vi "EAGLE Setup Screen V1.vi"() -> ()   [LabVIEW 2015]
panel:
  in  "AvgPulse":dbl(slide)=1.0 caption="Average Pulse\nEnergy [mJ]" min=0.0 max=1.0 step=0.1 scale=0.0..1.0
  out "Table Control":string[][](table)
  in  "EyeColor":enum32{"Dark", "Blue/Green"}(radio) caption="Eye Color"
  in  "EyeSelect":enum32{"Right Eye", "Left Eye"}(radio) caption="Treated Eye"
  in  "DisFromLimbus":dbl(slide)=1.0 caption="Distance From \nLimbus [um]" min=0.0 max=1.0 step=0.1 scale=0.0..1.0
  in  "TBetweenPulses":u8(slide)=4 caption="Time Between \nPulses [mSec]" min=4 max=10 step=1 scale=4.0..10.0
  in  "LaserShots":u8(slide)=1 caption="Number of \nLaser Shots" min=1 max=100 step=1 scale=1.0..100.0
  in  "ID":string caption="Patient ID"
  in  "TreatArea":enum32{"Upper 180", "Lower 180", "Full 360"}(radio) caption="Treatment Area"
  in  "SaveAs":bool
  in  "Save":bool
  in  "FillSetupList":bool
  in  "Treatment Setup":string(combo)
  in  "Done":bool
  # "Treatment Info"
  # "Patient Info"
  # "Treatment Summery"
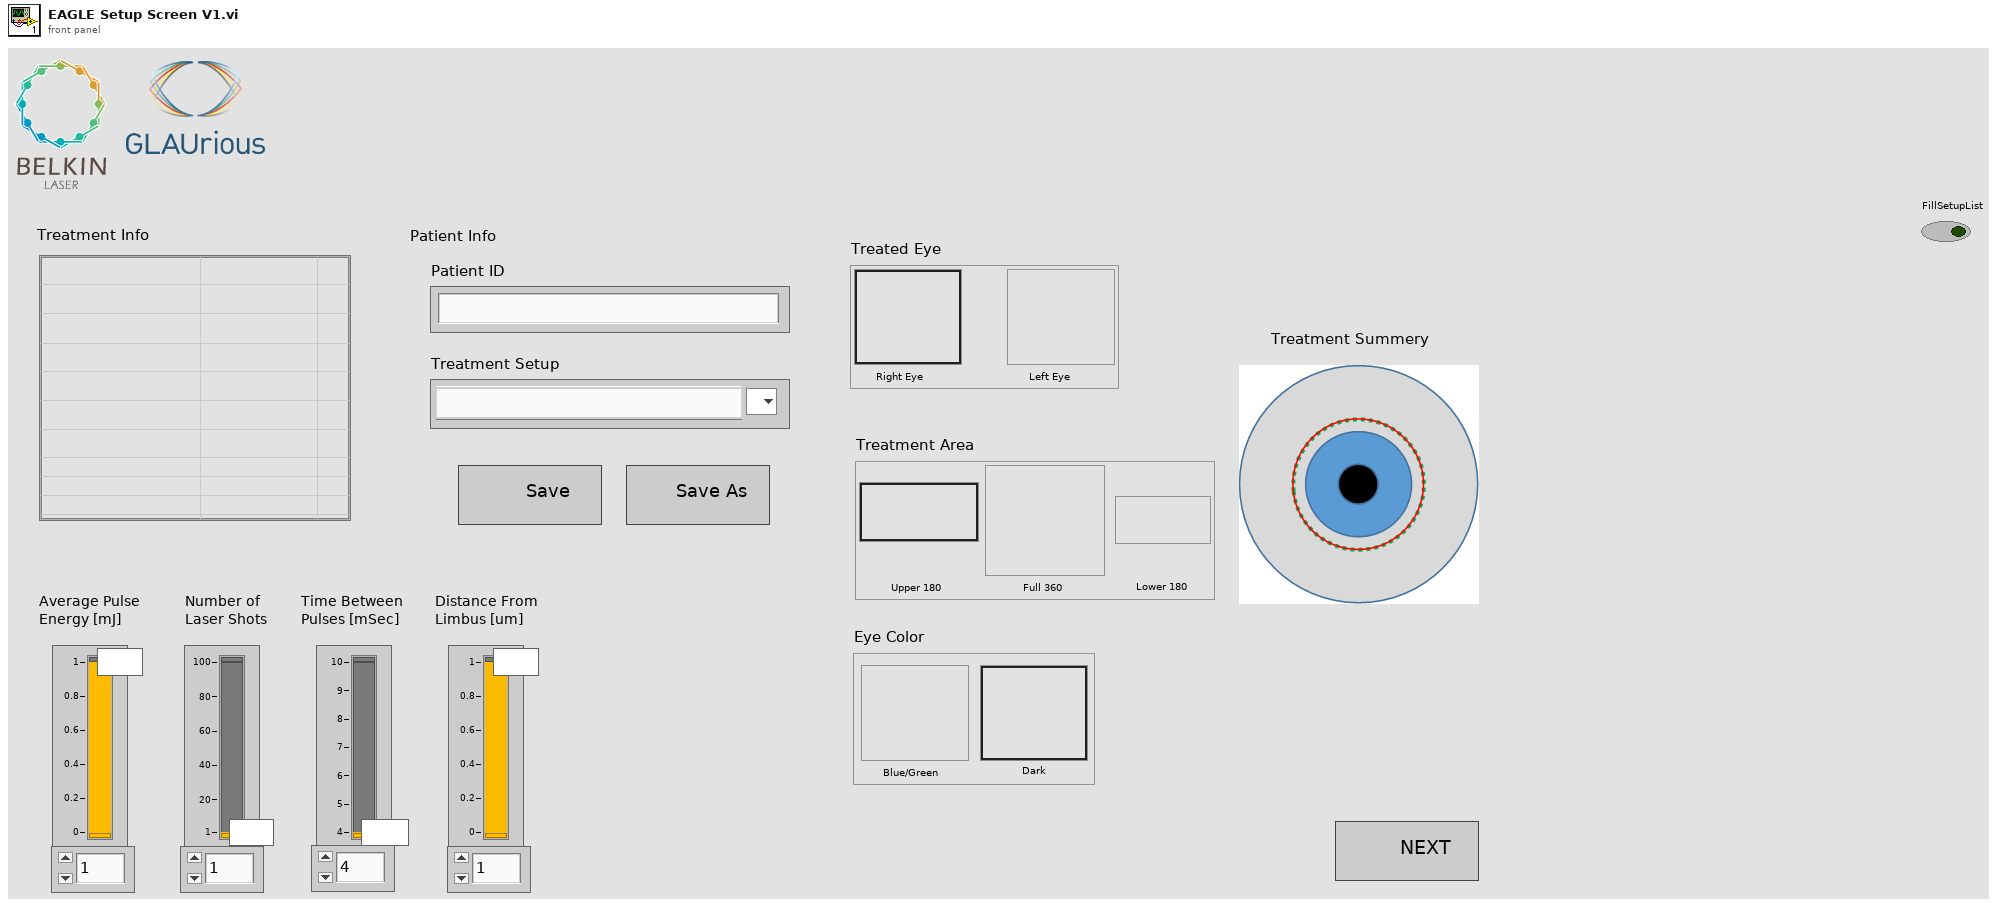
[diagram p1: front panel]
types:
  T1 = cluster{"EyeSelect":enum32{"Right Eye", "Left Eye"}, "TBetweenPulses":u8, "LaserShots":u8, "TreatArea":enum32{"Upper 180", "Lower 180", "Full 360"}, "DisFromLimbus":dbl, "ID":string, "EyeColor":enum32{"Dark", "Blue/Green"}, "AvgPulse":dbl}
  T2 = typedef "LVComboBoxStrsAndValuesArrayTypeDef.ctl" = cluster{"String":string, "Value":string}[]
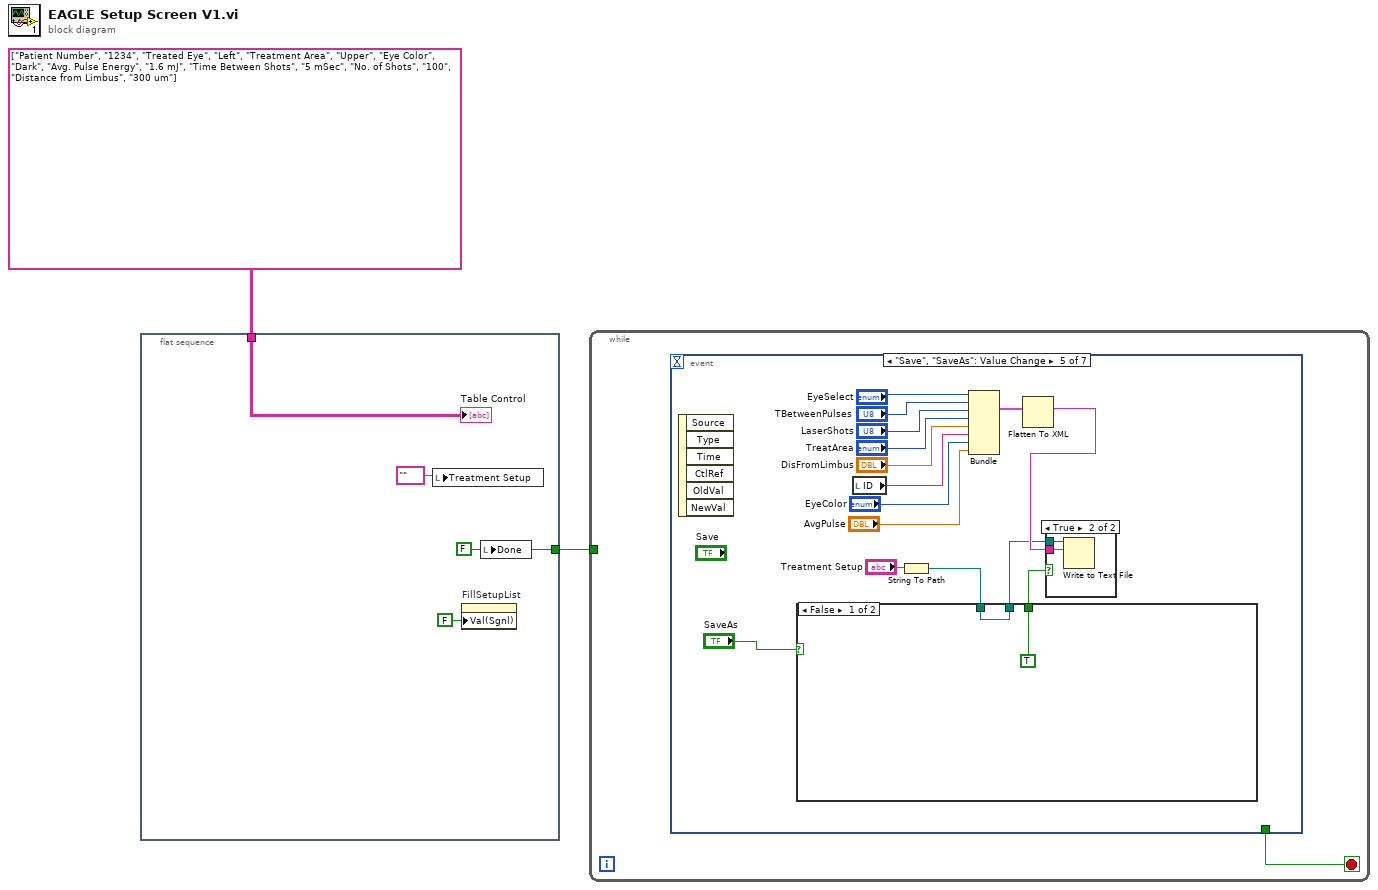
[diagram p0: block diagram]
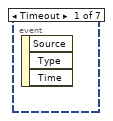
[diagram p2: hidden frame]
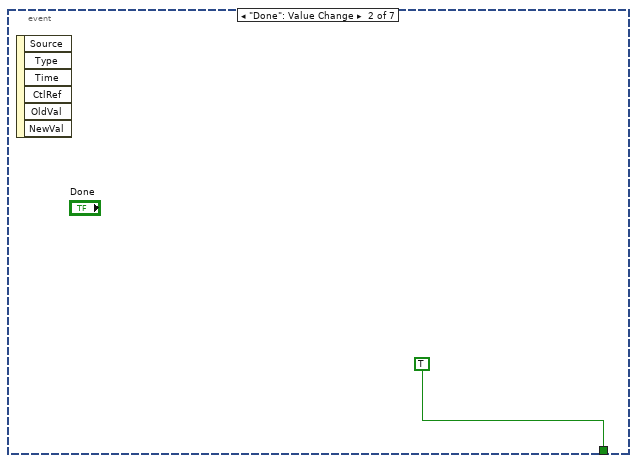
[diagram p3: hidden frame]
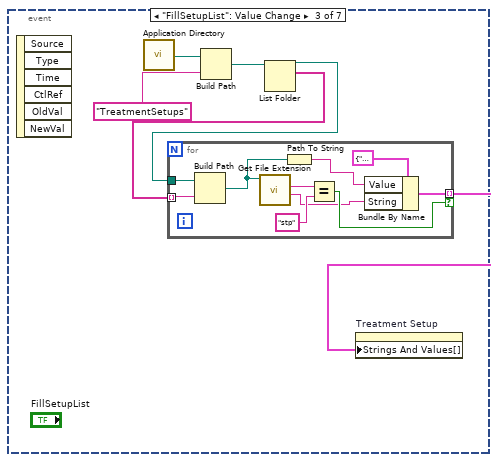
[diagram p4: hidden frame]
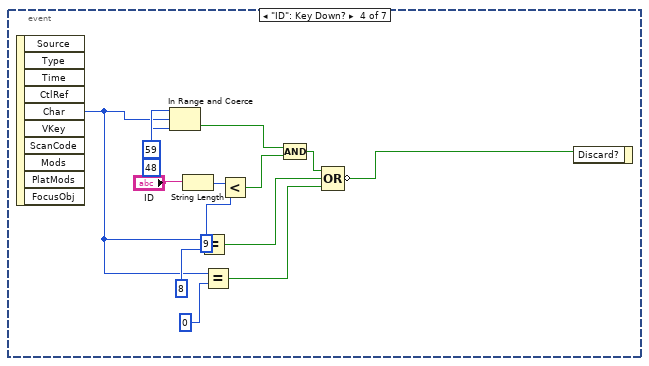
[diagram p5: hidden frame]
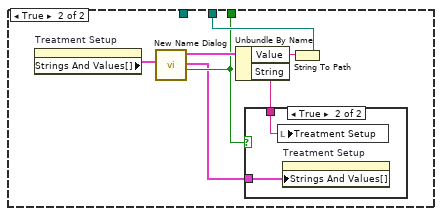
[diagram p7: hidden frame]
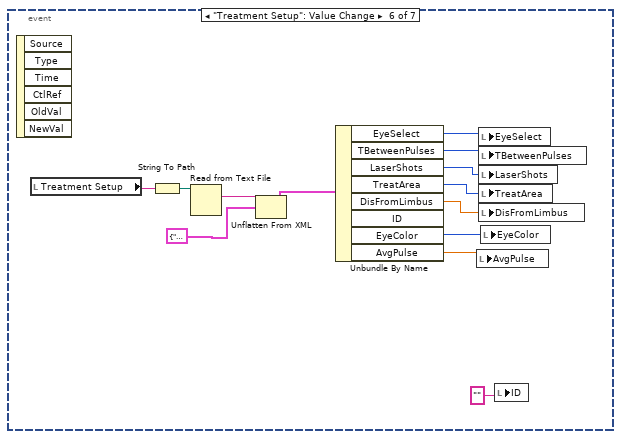
[diagram p9: hidden frame]
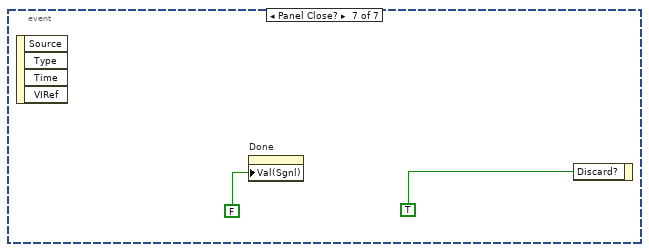
[diagram p10: hidden frame]
diagram:
  n1 = flat-sequence {
    tunnel: [w6] -> w2
    tunnel: string[][] [["Patient Number", "1234"], ["Treated Eye", "Left"], ["Treatment Area", "Upper"], ["Eye Color", "Dark"], ["Avg. Pulse Energy", "1.6 mJ"], ["Time Between Shots", "5 mSec"], ["No. of Shots", "100"], ["Distance from Limbus", "300 um"]] ("Table Control") -> [w3]
    frame #0 {
      w6 = FALSE ("Done")
      n2 = local write "Treatment Setup"("" ("Treatment Setup")) -> ()
      n3 = property on="FillSetupList" class="Bool (strict)"("Val(Sgnl)"=FALSE ("Value (Signaling)")) -> ()  [unwired: 2 in, 2 out]
      n4 = local write "Done"(w6) -> ()
      "Table Control" <- w3
    }
  }
  n5 = while {
    tunnel: w2 -> [_]
    stop <- w7 stop-if-true
    n6 = event shown="[4] \"Save\", \"SaveAs\": Value Change" {
      selector: _ -> [_ _ _ _ _ _ _]
      dyn-events: _ -> [_ _ _ _ _ _ _]
      timeout: _ -> [_ _ _ _ _ _ _]
      tunnel: [_ TRUE _ _ _ _ _] -> w7
      event Timeout {
        n7 = event-data() -> ()  [unwired: 1 in, 3 out]
      }
      event "Done": Value Change {
        n8 = event-data() -> ()  [unwired: 1 in, 6 out]
      }
      event "FillSetupList": Value Change {
        n9 = event-data() -> ()  [unwired: 1 in, 6 out]
        n10 = call <vilib>:"Application Directory.vi"() -> ("Application Directory"=w14:path)
        n11 = Build Path(base path=w14, name or relative path="TreatmentSetups") -> (appended path=w12:path)
        n12 = List Folder(path=w12) -> (path out=w10:path, filenames=w11:string[])  [unwired: 3 in, 2 out]
        n13 = for {
          tunnel: w11 -> [w19] mode=indexing
          tunnel: w10 -> [w24]
          tunnel: [w18] -> w9 mode=indexing if=w17
          n14 = Build Path(base path=w24, name or relative path=w19) -> (appended path=w22:path)
          n15 = call <vilib>:"Get File Extension.vi"("file"=w22) -> ("filename without extension"=w15:string, "lowercase file extension"=w16:string)  [unwired: 6 in, 3 out]
          n16 = Path To String(path=w22) -> (string=w20:string)
          n17 = Equal?(x=w16, y="stp") -> (x = y?=w17:bool)
          n18 = Bundle By Name(cluster=cluster{"String":string, "Value":string} {"String"="", "Value"=""}, "Value"=w20, "String"=w15) -> (w18:cluster{"String":string, "Value":string})
        }
        n19 = property on="Treatment Setup" class="CmbBox"("Strings And Values[]"=w9) -> ()  [unwired: 2 in, 2 out]
      }
      event "ID": Key Down? {
        n20 = event-data() -> ("Char"=w30:i16)  [unwired: 1 in, 9 out]
        n21 = In Range and Coerce(upper limit=i16 59, x=w30, lower limit=i16 48) -> (In Range?=w33:bool)  [unwired: 1 out]
        n22 = String Length(string="ID") -> (length=w35:i32)
        n23 = Equal?(x=w30, y=i16 8) -> (x = y?=w27:bool)
        n24 = Equal?(x=w30, y=i16 0) -> (x = y?=w26:bool)
        n25 = Less?(x=w35, y=9) -> (x < y?=w32:bool)
        n26 = Compound Arithmetic op=AND(w33, w32) -> (w28:bool)
        n27 = Compound Arithmetic op=OR(w28, w27, w26) -> (invert w25:bool)
        n28 = event-data("Discard?"=w25) -> ()  [unwired: 1 in, 1 out]
      }
      event "Save", "SaveAs": Value Change {
        n29 = event-data() -> ()  [unwired: 1 in, 6 out]
        n30 = local read "ID"() -> (w41:string)
        n31 = String To Path(string="Treatment Setup") -> (path=w44:path)
        n32 = case shown="False" "SaveAs" {
          tunnel: w44 -> [w57 _]
          tunnel: [w57 w61] -> w43
          tunnel: [TRUE w60] -> w42
          frame False {
          }
          frame True {
            n33 = property on="Treatment Setup" class="CmbBox"() -> ("Strings And Values[]"=w64:T2)  [unwired: 2 in, 2 out]
            n34 = call "New Name Dialog.vi"("Names"=w64) -> ("OK"=w60:bool, "NamesOut"=w59:cluster{"String":string, "Value":string}[], "NewName"=w63:cluster{"String":string, "Value":string})  [unwired: 8 in]
            n35 = Unbundle By Name(w63) -> ("Value"=w62:string, "String"=w58:string)
            n36 = case shown="True" w60 {
              tunnel: w59 -> [_ w66]
              tunnel: w58 -> [_ w65]
              frame False {
              }
              frame True {
                n37 = local write "Treatment Setup"(w65) -> ()
                n38 = property on="Treatment Setup" class="CmbBox"("Strings And Values[]"=w66) -> ()  [unwired: 2 in, 2 out]
              }
            }
            n39 = String To Path(string=w62) -> (path=w61:path)
          }
        }
        n40 = Bundle("EyeSelect"="EyeSelect", "TBetweenPulses"="TBetweenPulses", "LaserShots"="LaserShots", "TreatArea"="TreatArea", "DisFromLimbus"="DisFromLimbus", "ID"=w41, "EyeColor"="EyeColor", "AvgPulse"="AvgPulse") -> (w53:T1)  [unwired: 1 in]
        n41 = Flatten To XML(anything=w53) -> (xml string=w47:string)
        n42 = case shown="True" w42 {
          tunnel: w47 -> [_ w55]
          tunnel: w43 -> [_ w54]
          frame False {
          }
          frame True {
            n43 = Write to Text File(file (use dialog)=w54, text=w55) -> ()  [unwired: 2 in, 3 out]
          }
        }
      }
      event "Treatment Setup": Value Change {
        n44 = event-data() -> ()  [unwired: 1 in, 6 out]
        n45 = local read "Treatment Setup"() -> (w79:string)
        n46 = String To Path(string=w79) -> (path=w78:path)
        n47 = Read from Text File(file (use dialog)=w78) -> (text=w77:string)  [unwired: 3 in, 3 out]
        n48 = Unflatten From XML(xml string=w77, type=T1 {"EyeSelect"=enum."Right Eye", "TBetweenPulses"=0, "LaserShots"=0, "TreatArea"=enum."Upper 180", "DisFromLimbus"=0.0, "ID"="", "EyeColor"=enum."Dark", "AvgPulse"=0.0} ("output cluster")) -> (value=w76:T1)  [unwired: 1 in, 1 out]
        n49 = Unbundle By Name(w76) -> ("EyeSelect"=w75:enum32{"Right Eye", "Left Eye"}, "TBetweenPulses"=w74:u8, "LaserShots"=w73:u8, "TreatArea"=w72:enum32{"Upper 180", "Lower 180", "Full 360"}, "DisFromLimbus"=w71:dbl, "EyeColor"=w69:enum32{"Dark", "Blue/Green"}, "AvgPulse"=w67:dbl)  [unwired: 1 out]
        n50 = local write "AvgPulse"(w67) -> ()
        n51 = local write "EyeSelect"(w75) -> ()
        n52 = local write "TBetweenPulses"(w74) -> ()
        n53 = local write "LaserShots"(w73) -> ()
        n54 = local write "TreatArea"(w72) -> ()
        n55 = local write "DisFromLimbus"(w71) -> ()
        n56 = local write "EyeColor"(w69) -> ()
        n57 = local write "ID"("" ("ID")) -> ()
      }
      event Panel Close? {
        n58 = event-data() -> ()  [unwired: 1 in, 4 out]
        n59 = property on="Done" class="Bool (strict)"("Val(Sgnl)"=FALSE ("Value (Signaling)")) -> ()  [unwired: 2 in, 2 out]
        n60 = event-data("Discard?"=TRUE) -> ()  [unwired: 1 in, 1 out]
      }
    }
  }
